vi "XY Graph Save Plot.vi"(6 "Delimiter (TAB)":string="\t", 8 "Error In":errorcluster, 9 "Plot Index (-1: last plot)":i32=-1, 10 "File Path (empty: dialog)":path, 11 "XYGraph Ref":T1) -> (0 "Error Out":errorcluster, 1 "File Path":path, 2 "Plot Name":string, 3 "XYGraph Ref":T1, 4 "Cancelled":bool, 5 "Graph Name":string)   [LabVIEW 2021, in "XY Graph Add-Ons.lvlib"]
uses:
  XY Graph Add-Ons.lvlib
  XY Graph Refnum.ctl
  Files/Files.lvlib
  Arrays/Arrays.lvlib
  GUI/GUI.lvlib
  Strings/Strings.lvlib
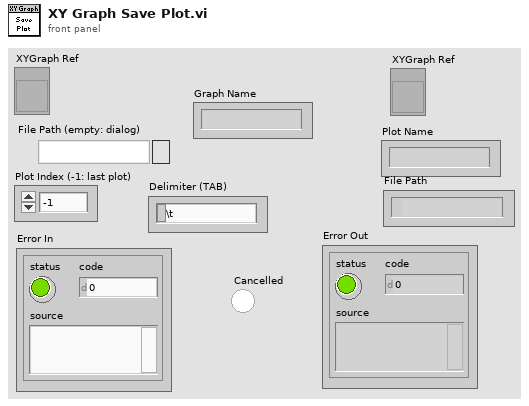
[diagram p1: front panel]
types:
  T1 = typedef "XY Graph Add-Ons.lvlib/XY Graph Refnum.ctl" = refnum<vi>
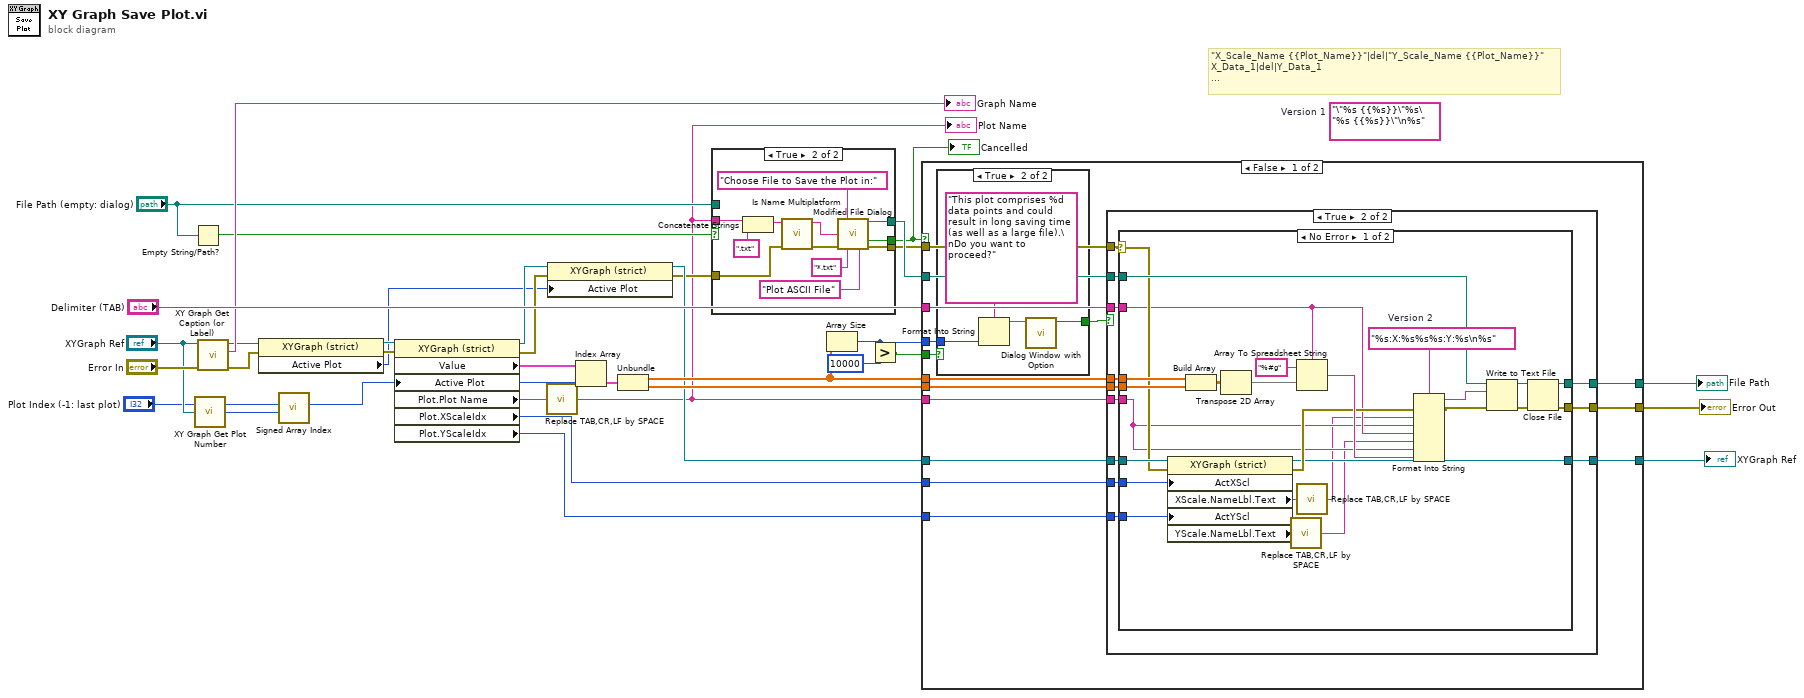
[diagram p0: block diagram]
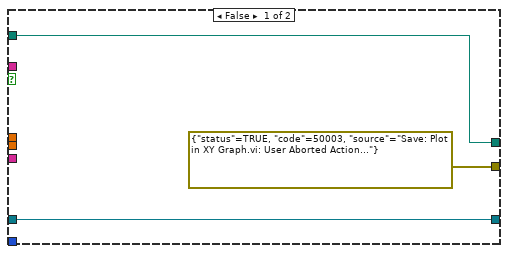
[diagram p3: hidden frame]
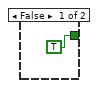
[diagram p5: hidden frame]
diagram:
  (unwired) "\"%s {{%s}}\"%s\"%s {{%s}}\"\n%s"  # Version 1
  # "\"X_Scale_Name {{Plot_Name}}\"|del|\"Y_Scale_Name {{Plot_Name}}\"\nX_Data_1|del|Y_Data_1\n..."
  n1 = Empty String/Path?(string/path="File Path (empty: dialog)") -> (empty?=w3:bool)
  n2 = call "XY Graph Get Plot Number.vi"("XYGraph"="XYGraph Ref") -> ("# Plots"=w10:i32)  [unwired: 8 in]
  n3 = call "XY Graph Get Caption (or Label).vi"("error in (no error)"="Error In", "XYGraph in"="XYGraph Ref") -> ("error out"=w14:errorcluster, "Caption (or Label) Text"=→"Graph Name":string, "XYGraph out"=w16:T1)  [unwired: 7 in]
  n4 = property class="XYGraph (strict)"(reference=w16, error in=w14) -> (reference out=w15:T1, error out=w13:errorcluster, "Active Plot"=w4:u32)
  n5 = call "Signed Array Index.vi"("Array Size"=w10, "Array Index in"="Plot Index (-1: last plot)") -> ("Array Index out"=w9:i32)  [unwired: 9 in]
  n6 = property class="XYGraph (strict)"(reference=w15, error in=w13, "Active Plot"=w9) -> (reference out=w8:T1, error out=w6:errorcluster, "Value"=w35:cluster{"X Array":dbl[], "Y Array":dbl[]}[], "Plot.Plot Name"=w30:string, "Plot.XScaleIdx"=w33:u32, "Plot.YScaleIdx"=w32:u32)
  n7 = call "Replace TAB,CR,LF by SPACE.vi"("String"=w30) -> ("String with replacements"=w1:string)  [unwired: 8 in]
  "Plot Name" <- w1
  n8 = property class="XYGraph (strict)"(reference=w8, error in=w6, "Active Plot"=w4) -> (reference out=w7:T1, error out=w5:errorcluster)
  n9 = Index Array(array=w35, index=w9) -> (element=w34:cluster{"X Array":dbl[], "Y Array":dbl[]})
  n10 = Unbundle(w34) -> ("X Array"=w24:dbl[], "Y Array"=w31:dbl[])
  n11 = case shown="True" w3 {
    tunnel: w1 -> [_ w49]
    tunnel: [w37 w48] -> w29
    tunnel: [w36 w47] -> w26
    tunnel: [_ w42] -> w17
    tunnel: w5 -> [w36 w38]
    tunnel: "File Path (empty: dialog)" -> [w37 _]
    frame False {
    }
    frame True {
      n12 = Concatenate Strings(w49, ".txt" ("string")) -> (w45:string)
      n13 = call <vilib>:"Is Name Multiplatform.vi"("error in (no error)"=w38, "filename"=w45) -> ("error out"=w44:errorcluster, "suggested filename"=w43:string)  [unwired: 5 in, 3 out]
      n14 = call "Modified File Dialog.vi"("prompt"="Choose File to Save the Plot in:", "suggested filename"=w43, "error in (no error)"=w44, "pattern"="*.txt" ("pattern (all files)"), "pattern label"="Plot ASCII File") -> ("selected path"=w48:path, "Cancelled"=w42:bool, "error out"=w47:errorcluster)  [unwired: 7 in, 1 out]
    }
  }
  "Cancelled" <- w17
  n15 = Array Size(array=w24) -> (size(s)=w22:i32)
  n16 = Greater?(x=w22, y=10000) -> (0:w21:bool)
  n17 = case shown="False" w17 {
    tunnel: w7 -> [w64 w115]
    tunnel: w33 -> [w63 _]
    tunnel: w32 -> [w62 _]
    tunnel: w31 -> [w61 _]
    tunnel: w1 -> [w60 _]
    tunnel: w29 -> [w59 w113]
    tunnel: [w58 w114] -> w28
    tunnel: [w57 w113] -> w27
    tunnel: w26 -> [w56 w114]
    tunnel: "Delimiter (TAB)" -> [w55 _]
    tunnel: w24 -> [w54 _]
    tunnel: w22 -> [w53 _]
    tunnel: w21 -> [w52 _]
    tunnel: [w50 w115] -> w20
    frame False {
      n18 = case shown="True" w52 {
        tunnel: w53 -> [_ w111]
        tunnel: [TRUE ("T button?") w109] -> w51
        frame False {
        }
        frame True {
          n19 = Format Into String(format string="This plot comprises %d data points and could result in long saving time (as well as a large file).\nDo you want to proceed?", w111) -> (resulting string=w110:string)  [unwired: 2 in, 1 out]
          n20 = call "Dialog Window with Option.vi"("Message"=w110) -> ("OK?"=w109:bool)  [unwired: 8 in, 2 out]
        }
      }
      n21 = case shown="True" w51 {
        tunnel: w64 -> [w65 w79]
        tunnel: w63 -> [_ w78]
        tunnel: w62 -> [_ w77]
        tunnel: w61 -> [_ w76]
        tunnel: w60 -> [_ w75]
        tunnel: w59 -> [w66 w74]
        tunnel: [errorcluster {"status"=TRUE, "code"=50003, "source"="Save: Plot in XY Graph.vi: User Aborted Action..."} ("error IO") w73] -> w58
        tunnel: [w66 w72] -> w57
        tunnel: w56 -> [_ w71]
        tunnel: w55 -> [_ w70]
        tunnel: w54 -> [_ w69]
        tunnel: [w65 w68] -> w50
        frame False {
        }
        frame True {
          n22 = case shown="No Error" w71 {
            selector: w71 -> [w87 w107]
            tunnel: w79 -> [w105 w106]
            tunnel: w78 -> [w104 _]
            tunnel: w77 -> [w103 _]
            tunnel: w69 -> [w102 _]
            tunnel: w76 -> [w101 _]
            tunnel: w75 -> [w84 _]
            tunnel: w74 -> [w91 _]
            tunnel: [w85 w107] -> w73
            tunnel: [w83 _] -> w72
            tunnel: w70 -> [w86 _]
            tunnel: [w82 w106] -> w68
            frame No Error {
              w97 = "%s:X:%s%s%s:Y:%s\n%s"  # Version 2
              n23 = property class="XYGraph (strict)"(reference=w105, error in=w87, "ActXScl"=w104, "ActYScl"=w103) -> (reference out=w82:T1, error out=w93:errorcluster, "XScale.NameLbl.Text"=w96:string, "YScale.NameLbl.Text"=w95:string)
              n24 = Build Array(w102, w101) -> (w100:dbl[][])
              n25 = Transpose 2D Array(2D array=w100) -> (transposed array=w99:dbl[][])
              n26 = call "Replace TAB,CR,LF by SPACE.vi"("String"=w95) -> ("String with replacements"=w80:string)  [unwired: 8 in]
              n27 = Array To Spreadsheet String(delimiter (Tab)=w86, array=w99, 3:"%#g" ("format string")) -> (spreadsheet string=w94:string)
              n28 = call "Replace TAB,CR,LF by SPACE.vi"("String"=w96) -> ("String with replacements"=w81:string)  [unwired: 8 in]
              n29 = Format Into String(format string=w97, error in=w93, w81, w84, w86, w80, w84, w94) -> (resulting string=w92:string, error out=w90:errorcluster)  [unwired: 1 in]
              n30 = Write to Text File(file (use dialog)=w91, text=w92, error in=w90) -> (refnum out=w89:refnum<file>, error out=w88:errorcluster)  [unwired: 1 in, 1 out]
              n31 = Close File(refnum=w89, error in=w88) -> (path=w83:path, error out=w85:errorcluster)
            }
            frame Error {
            }
          }
        }
      }
    }
    frame True {
    }
  }
  "Error Out" <- w28
  "File Path" <- w27
  "XYGraph Ref" <- w20
